vi "XML Write to FOFB Controller.vi"(5 "Password":string, 7 "User":string, 8 "error in (no error)":errorcluster, 10 "FOFB Parameters":T1, 11 "FOFB-Controller IP Address in":string) -> (0 "error out":errorcluster)   [LabVIEW 2011, in "XML VIs.lvlib"]
uses:
  XML VIs.lvlib
  Types Definitions/Type FOFB Parameters.ctl
  Types Definitions/Type Network Configuration.ctl
  Types Definitions/Type FA Configuration.ctl
  Types Definitions/Type Response Matrix Measurement Configuration.ctl
  Types Definitions/Type Correction Algorithm Configuration.ctl
  Types Definitions/Type Acquisition Network Configuration.ctl
  Types Definitions/Type Actuation Network Configuration.ctl
  <vilib>/addons/internet/NI_InternetTK_FTP_VIs.lvlib
  Type Definitions.lvlib
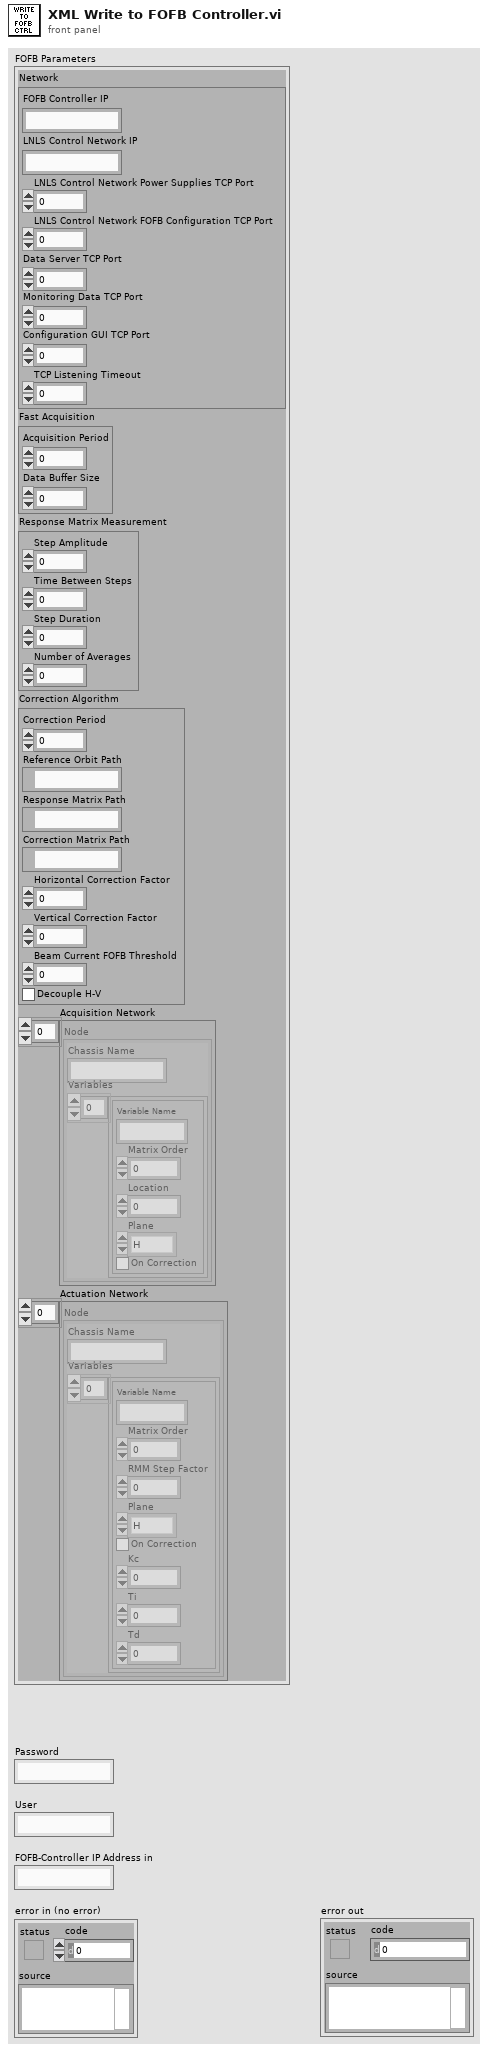
[diagram p1: front panel]
types:
  T1 = typedef "Type Definitions.lvlib/Type FOFB Parameters.ctl" = cluster{"Network":T2, "Fast Acquisition":T3, "Response Matrix Measurement":T4, "Correction Algorithm":T5, "Acquisition Network":T6, "Actuation Network":T7}
  T2 = typedef "Type Definitions.lvlib/Type Network Configuration.ctl" = cluster{"FOFB Controller IP":string, "LNLS Control Network IP":string, "LNLS Control Network Power Supplies TCP Port":u16, "LNLS Control Network FOFB Configuration TCP Port":u16, "Data Server TCP Port":u16, "Monitoring Data TCP Port":u16, "Configuration GUI TCP Port":u16, "TCP Listening Timeout":i32}
  T3 = typedef "Type Definitions.lvlib/Type FA Configuration.ctl" = cluster{"Acquisition Period":u32, "Data Buffer Size":u32}
  T4 = typedef "Type Definitions.lvlib/Type Response Matrix Measurement Configuration.ctl" = cluster{"Step Amplitude":dbl, "Time Between Steps":u32, "Step Duration":u32, "Number of Averages":u32}
  T5 = typedef "Type Definitions.lvlib/Type Correction Algorithm Configuration.ctl" = cluster{"Correction Period":u32, "Reference Orbit Path":path, "Response Matrix Path":path, "Correction Matrix Path":path, "Horizontal Correction Factor":dbl, "Vertical Correction Factor":dbl, "Beam Current FOFB Threshold":dbl, "Decouple H-V":bool}
  T6 = typedef "Type Definitions.lvlib/Type Acquisition Network Configuration.ctl" = cluster{"Chassis Name":string, "Variables":cluster{"Variable Name":string, "Matrix Order":u32, "Location":dbl, "Plane":enum8{"H", "V"}, "On Correction":bool}[]}[]
  T7 = typedef "Type Definitions.lvlib/Type Actuation Network Configuration.ctl" = cluster{"Chassis Name":string, "Variables":cluster{"Variable Name":string, "Matrix Order":u32, "RMM Step Factor":dbl, "Plane":enum8{"H", "V"}, "On Correction":bool, "Kc":dbl, "Ti":dbl, "Td":dbl}[]}[]
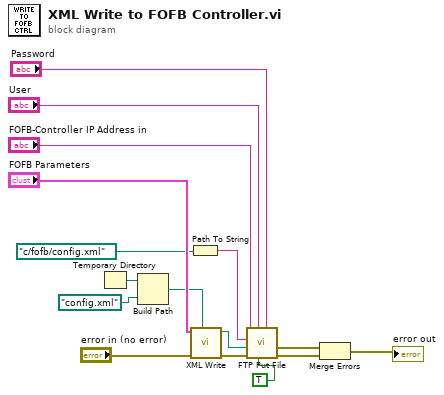
[diagram p0: block diagram]
diagram:
  n1 = Temporary Directory() -> (w5:path)
  n2 = Build Path(base path=w5, name or relative path=path "config.xml") -> (appended path=w12:path)
  n3 = Path To String(path=path "c:/fofb/config.xml") -> (string=w8:string)
  n4 = call "XML Write.vi"("XML File Path Write"=w12, "Error In"="error in (no error)", "FOFB Parameters"="FOFB Parameters") -> ("Error Out"=w15:errorcluster, "XML File Path Out"=w13:path)  [unwired: 7 in]
  n5 = call <vilib>:"FTP Put File.vi"("password"="Password", "binary (F)"=TRUE, "user"="User", "error in (no error)"=w15, "local path"=w13, "remote path"=w8, "host"="FOFB-Controller IP Address in") -> ("error out"=w2:errorcluster, "file error"=w3:errorcluster)  [unwired: 3 in]
  n6 = Merge Errors(w3, w2) -> (→"error out":errorcluster)
